vi "Hatch Panel Intake.vi"   [LabVIEW 2018]
uses:
  <vilib>/Rock Robotics/WPI/Solenoid/WPI_SolenoidChannel.ctl
  <vilib>/Rock Robotics/WPI/Solenoid/WPI_SolenoidValue.ctl
  <vilib>/Rock Robotics/WPI/Solenoid/WPI_SolenoidOpenSingle.vi
  Hatch Panel Intake Global.vi
  <vilib>/Rock Robotics/WPI/Solenoid/WPI_SolenoidSetEnum.vi
types:
  T1 = typedef "WPI_SolenoidChannel.ctl" = enum8{"Solenoid 0", "Solenoid 1", "Solenoid 2", "Solenoid 3", "Solenoid 4", "Solenoid 5", "Solenoid 6", "Solenoid 7", "Invalid"}
  T2 = typedef "WPI_SolenoidDevRef.ctl" = cluster{"DevStatus":errorcluster, "Pneumatics Control Module":u8, "Forward Solenoid Channel":T1, "Reverse Solenoid Channel":T1}
  T3 = typedef "WPI_SolenoidValue.ctl" = enum16{"Off", "On", "Forward", "Reverse"}
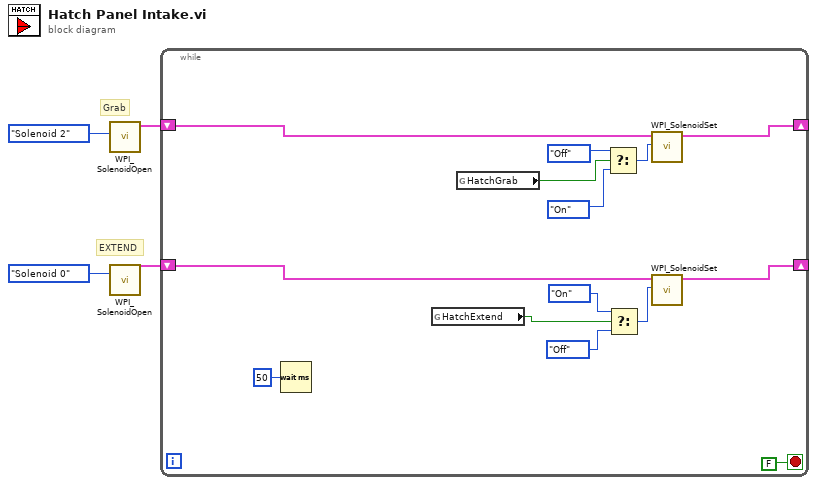
[diagram p0: block diagram]
diagram:
  # "EXTEND"
  # "Grab"
  n1 = call-poly <vilib>:"WPI_SolenoidOpen.vi"("Solenoid Channel"=WPI_SolenoidChannel."Solenoid 2" ("Forward Solenoid Channel")) -> ("SolenoidDevRef"=w1:T2)  [unwired: 9 in, 1 out]
  n2 = call-poly <vilib>:"WPI_SolenoidOpen.vi"("Solenoid Channel"=WPI_SolenoidChannel."Solenoid 0" ("Forward Solenoid Channel")) -> ("SolenoidDevRef"=w4:T2)  [unwired: 9 in, 1 out]
  n3 = while {
    shift-right: [w15] -> _
    shift-left: w1 -> [w16]
    shift-right: [w14] -> _
    shift-left: w4 -> [w17]
    stop <- FALSE stop-if-true
    n4 = Wait (ms)(milliseconds to wait=u32 50) -> ()  [unwired: 1 out]
    n5 = global read "Hatch Panel Intake Global.vi" "HatchExtend"() -> (w5:bool)
    n6 = global read "Hatch Panel Intake Global.vi" "HatchGrab"() -> (w6:bool)
    n7 = Select(t=WPI_SolenoidValue."Off" ("Value"), s=w6, f=WPI_SolenoidValue."On" ("Value")) -> (s? t:f=w8:T3)
    n8 = Select(t=WPI_SolenoidValue."On" ("Value"), s=w5, f=WPI_SolenoidValue."Off" ("Value")) -> (s? t:f=w11:T3)
    n9 = call-poly <vilib>:"WPI_SolenoidSet.vi"("Value"=w8, "SolenoidDevRef"=w16) -> ("SolenoidDevRef"=w15:T2)  [unwired: 8 in, 1 out]
    n10 = call-poly <vilib>:"WPI_SolenoidSet.vi"("Value"=w11, "SolenoidDevRef"=w17) -> ("SolenoidDevRef"=w14:T2)  [unwired: 8 in, 1 out]
  }
